vi "MTM2_getSample_displacementSensors.vi"(8 "error in (no error)":errorcluster, 11 "displacementSensors_Ctl":T1={"private_rcvStamp"=0.0, "thetaZ[6]"=[0.0, 0.0, 0.0, 0.0, 0.0, 0.0], "deltaZ[6]"=[0.0, 0.0, 0.0, 0.0, 0.0, 0.0]}) -> (0 "error out":errorcluster, 2 "function return":i32, 3 "displacementSensors_Ctl out":T1)   [LabVIEW 2018, in "SALLV_MTM2.lvlib"]
doc: "int MTM2_shm_getSample_displacementSensorsLV(MTM2_displacementSensorsLV *displacementSensors_Ctl );"
uses:
  DataTypes/displacementSensors.ctl
  SALLV_MTM2.lvlib
  SALLV_MTM2.so
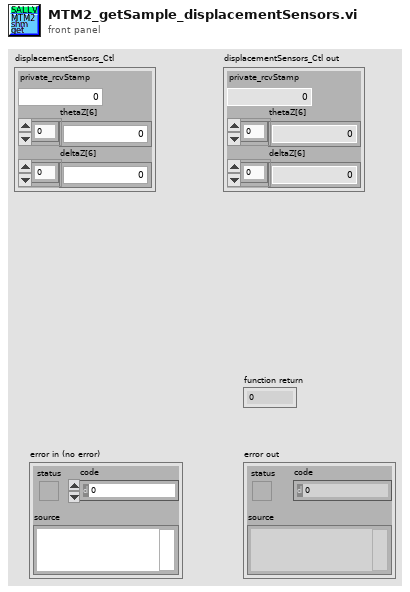
[diagram p1: front panel]
types:
  T1 = typedef "SALLV_MTM2.lvlib/displacementSensors.ctl" = cluster{"private_rcvStamp":dbl, "thetaZ[6]":dbl[], "deltaZ[6]":dbl[]}
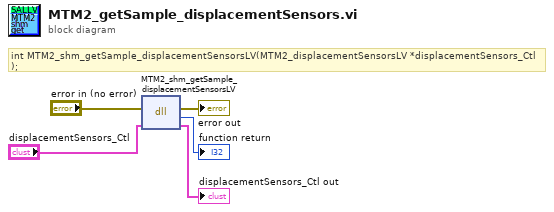
[diagram p0: block diagram]
diagram:
  # "int MTM2_shm_getSample_displacementSensorsLV(MTM2_displacementSensorsLV *displacementSensors_Ctl );"
  n1 = dll-call lib="home/ttsai/Documents/salLabviewApi/SALLV_MTM2/SALLV_MTM2.*" fn="MTM2_shm_getSample_displacementSensorsLV"(error in="error in (no error)", "displacementSensors_Ctl"="displacementSensors_Ctl") -> (error out=→"error out":errorcluster, →"function return":i32, "displacementSensors_Ctl"=→"displacementSensors_Ctl out":T1)  [unwired: 2 in, 1 out]
